vi "Introspection Core.vi"(8 "error in (no error)":errorcluster, 11 "LS218 in":refnum<class "LS218.lvclass">) -> (0 "error out":errorcluster, 2 "CS++Messages":refnum<class "Message.lvclass">[](array[class]), 3 "LS218 out":refnum<class "LS218.lvclass">)   [LabVIEW 2016, in "LS218.lvlib" / "LS218.lvclass"]
doc: "This vi delivers a list with all messages this actor reacts to. \n\nNote that all inherited classes have to overwrite it."
uses:
  LS218.lvclass
  <vilib>/ActorFramework/Message/Message.lvclass
  LS218 Messages/Write calibration curves to instruments Msg/Write calibration curves to instruments Msg.lvclass
  C:/Program Files (x86)/National Instruments/LabVIEW 2016/vi.lib/ActorFramework/Message/Message.lvclass
  LS218 Messages/Configure Alarms Msg/Configure Alarms Msg.lvclass
  LS218 Messages/Configure Relays Msg/Configure Relays Msg.lvclass
  LS218 Messages/Log Data Msg/Log Data Msg.lvclass
  LS218 Messages/Reset Alarms Msg/Reset Alarms Msg.lvclass
  LS218 Messages/Reset Min-Max Msg/Reset Min-Max Msg.lvclass
  LS218 Messages/Read All Sensor Data Msg/Read All Sensor Data Msg.lvclass
  LS218 Messages/Write Single Calibration Curve to Instrument Msg/Write Single Calibration Curve to Instrument Msg.lvclass
  CSPP_Core/Actors/CS++DeviceActor/CS++DeviceActor.lvclass
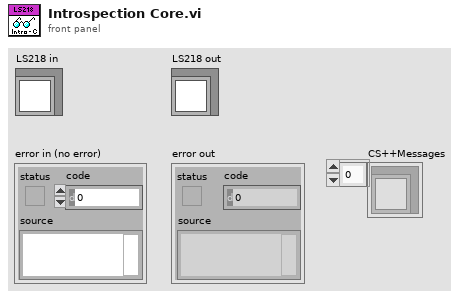
[diagram p1: front panel]
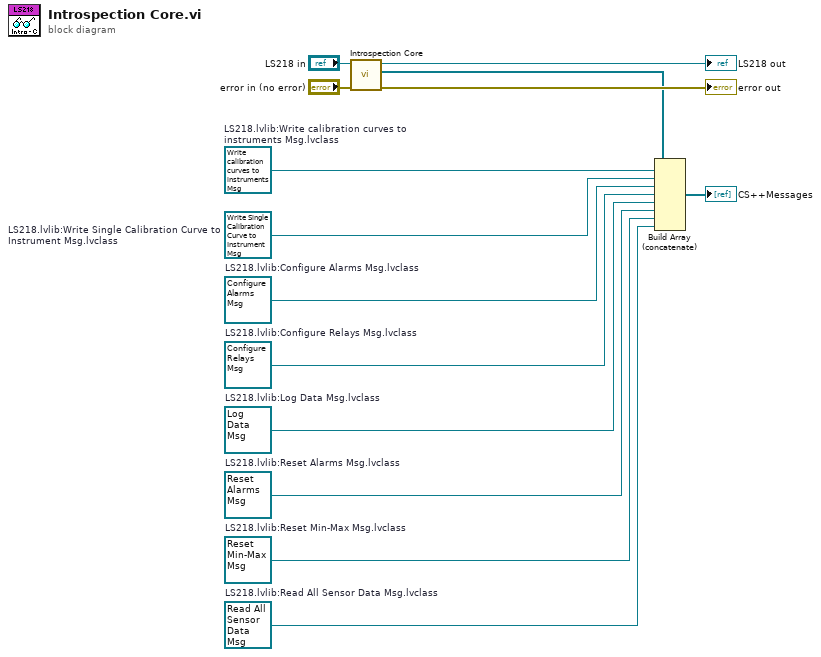
[diagram p0: block diagram]
diagram:
  w1 = refnum<class "Write Single Calibration Curve to Instrument Msg.lvclass"> refnum  # LS218.lvlib:Write Single Calibration Curve to Instrument Msg.lvclass
  w2 = refnum<class "Read All Sensor Data Msg.lvclass"> refnum  # LS218.lvlib:Read All Sensor Data Msg.lvclass
  w3 = refnum<class "Reset Min-Max Msg.lvclass"> refnum  # LS218.lvlib:Reset Min-Max Msg.lvclass
  w4 = refnum<class "Reset Alarms Msg.lvclass"> refnum  # LS218.lvlib:Reset Alarms Msg.lvclass
  w5 = refnum<class "Log Data Msg.lvclass"> refnum  # LS218.lvlib:Log Data Msg.lvclass
  w6 = refnum<class "Configure Relays Msg.lvclass"> refnum  # LS218.lvlib:Configure Relays Msg.lvclass
  w7 = refnum<class "Configure Alarms Msg.lvclass"> refnum  # LS218.lvlib:Configure Alarms Msg.lvclass
  w10 = refnum<class "Write calibration curves to instruments Msg.lvclass"> refnum  # LS218.lvlib:Write calibration curves to instruments Msg.lvclass
  n1 = call-parent "Introspection Core.vi"("error in (no error)"="error in (no error)", "CS++DeviceActor in"="LS218 in") -> ("error out"=→"error out":errorcluster, "CS++Messages"=w9:refnum<class "Message.lvclass">[], "CS++DeviceActor out"=→"LS218 out":refnum<class "LS218.lvclass">)  [unwired: 7 in]
  n2 = Build Array (concatenate)(w9, w10, w1, w7, w6, w5, w4, w3, w2) -> (→"CS++Messages":refnum<class "Message.lvclass">[])
